vi "SQLExecute.vi"(4 "error in (no error)":errorcluster, 7 "InputHandle":i32) -> (0 "error out":errorcluster, 3 "OutputHandle":i32)   [LabVIEW 2011]
doc: "Execute la requête spécifiée par le lien et préalablemet chargée"
uses:
  Odbc32.dll
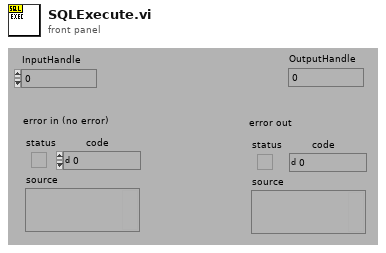
[diagram p1: front panel]
types:
  T1 = enum16{"NOPE", "SQL_HANDLE_ENV", "SQL_HANDLE_DBC", "SQL_HANDLE_STMT", "SQL_HANDLE_DESC"}
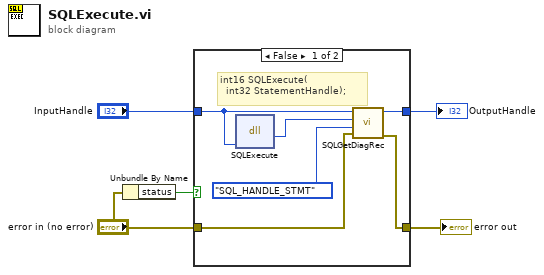
[diagram p0: block diagram]
diagram:
  n1 = Unbundle By Name("error in (no error)") -> ("status"=w1:bool)
  n2 = case shown="False" w1 {
    tunnel: "InputHandle" -> [w10 w13]
    tunnel: [w9 w13] -> w4
    tunnel: [w8 w12] -> w3
    tunnel: "error in (no error)" -> [w7 w12]
    frame False {
      # "int16 SQLExecute(\n  int32 StatementHandle);"
      n3 = dll-call lib="Odbc32.dll" fn="SQLExecute"("StatementHandle"=w10) -> (w11:i16)  [unwired: 4 in, 2 out]
      n4 = call "SQLGetDiagRec.vi"("error in (no error)"=w7, "HandleType"=T1."SQL_HANDLE_STMT", "Status (SQL_SUCCESS=0)"=w11, "Input Handle"=w10) -> ("error out"=w8:errorcluster, "Output Handle"=w9:i32)  [unwired: 2 out]
    }
    frame True {
    }
  }
  "OutputHandle" <- w4
  "error out" <- w3
